vi "Pulse Generator 2.vi"() -> ()   [LabVIEW 2012]
uses:
  <vilib>/DAQmx/read.llb/DAQmx Read (Digital 1D Bool 1Chan 1Samp).vi
  <vilib>/DAQmx/create/channels.llb/DAQmx Create Channel (DI-Digital Input).vi
  <vilib>/DAQmx/miscellaneous.llb/DAQmx Fill In Error Info.vi
  <vilib>/Utility/file.llb/Write To Spreadsheet File (DBL).vi
panel:
  out "Track":bool=TRUE
  in  "ref?":bool=TRUE
  in  "load":bool
  in  "MW Delay":dbl=5e-08
  in  "Sig/Ref pause":dbl=7e-07
  in  "Tab Control":T1(tab)=enum."FLIM"
  in  "Rate (Hz)":dbl=1000.0
  in  "Pulse MW":bool=TRUE
  in  "Pulse Laser":bool
  in  "Delay Blocks":u16=4
  in  "Divide By":u16(ring) items=["1", "8", "16", "32"]
  in  "MW width Min":dbl=2e-08
  in  "MW width step size":dbl=5e-09
  in  "MW width Max":dbl=5e-07
  in  "Tau step size":dbl
  in  "Tau max":dbl
  in  "Tau min":dbl
  in  "Rabi Frequency":dbl
  in  "Pulse offset 2":dbl
  in  "Rabi Frequency":dbl
  in  "Tau max":dbl
  in  "Tau min":dbl
  in  "Tau step size":dbl
  in  "Equal Pulse length":bool
  in  "Pulse offset":dbl
  in  "Tau":dbl
  in  "Rabi Frequency  2":dbl
  in  "Tau' max 2":dbl
  in  "Tau' min 2":dbl
  in  "Tau' step size 2":dbl
  in  "Rabi Frequency":dbl
  in  "Tau min":dbl
  in  "Tau max":dbl
  in  "Tau step size":dbl
  in  "No. Pi Pulses":i32
  in  "Pulse offset":dbl
  in  "0->+?":bool
  in  "AOM Rest time":dbl=2e-06
  in  "Signal delay":dbl=1.1e-06
  in  "N Loop":i32=10000
  in  "APD signal width":dbl=5e-07
  out "Run":bool=TRUE
  out "Scan size":i32
  in  "file path (dialog if empty)":path=path "C:/Users/Ouyang Group/Documents/Data/12-5-13/current"
  in  "AOM Pulse length":dbl=2e-06
  in  "Path to spinapi.dll":path=path "C:/SpinCore/SpinAPI/dll/spinapi64.dll"
  in  "stop":bool
  in  "start/restart":bool
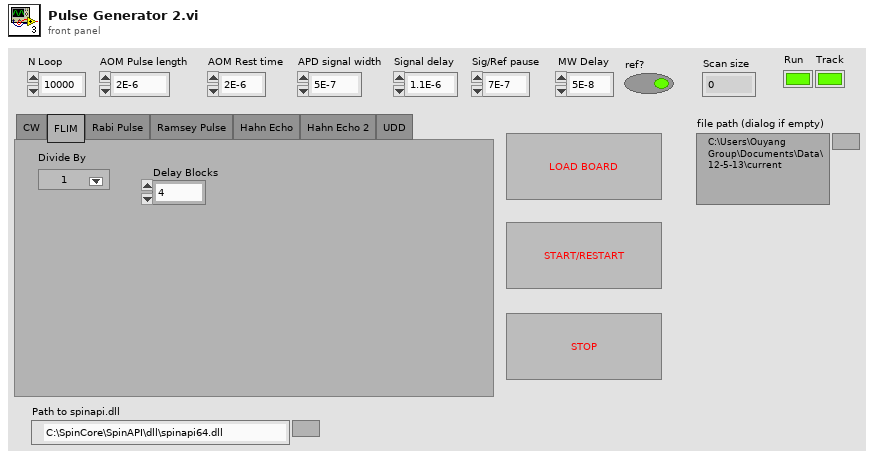
[diagram p1: front panel]
types:
  T1 = enum32{"CW", "FLIM", "Rabi Pulse", "Ramsey Pulse", "Hahn Echo", "Hahn Echo 2", "UDD"}
  T2 = enum16{"Pulse Program", "Frequency Registers", "TX Phase Registers", "RX Phase Registers"}
  T3 = cluster{"Instruct Data":i32, "Op Code":i32, "Flags":bool[], "Comments":string, "Time (s)":dbl}
  T4 = cluster{"Instruct Data":i32, "Op Code":i32, "Flags":bool[], "Comments":string, "Time (s)":dbl}[]
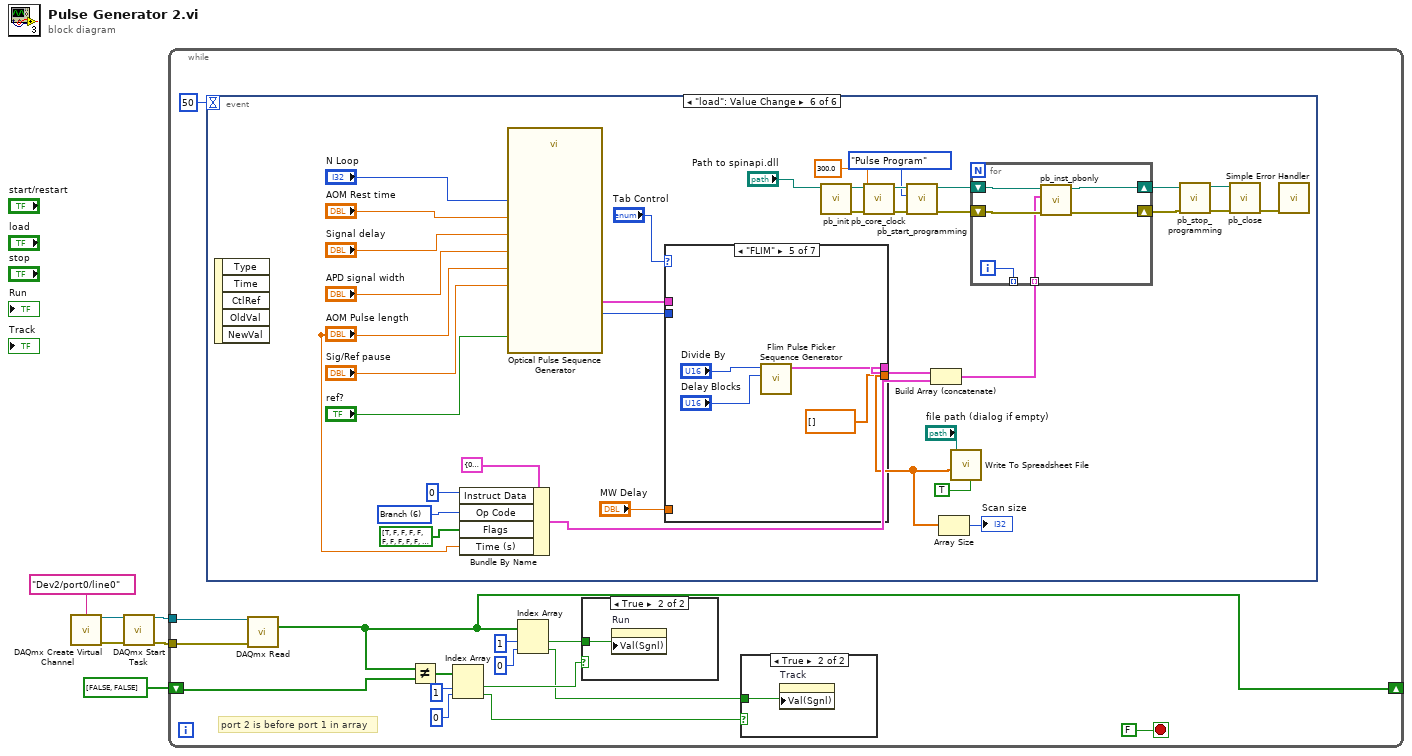
[diagram p0: block diagram]
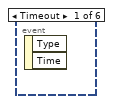
[diagram p3: hidden frame]
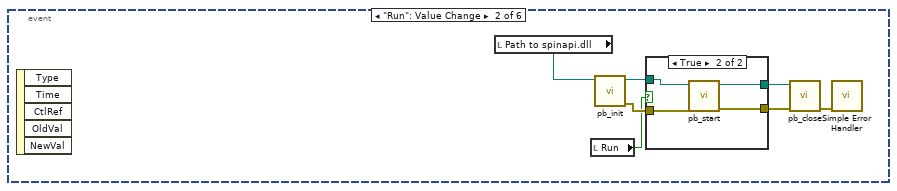
[diagram p4: hidden frame]
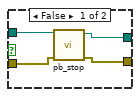
[diagram p5: hidden frame]
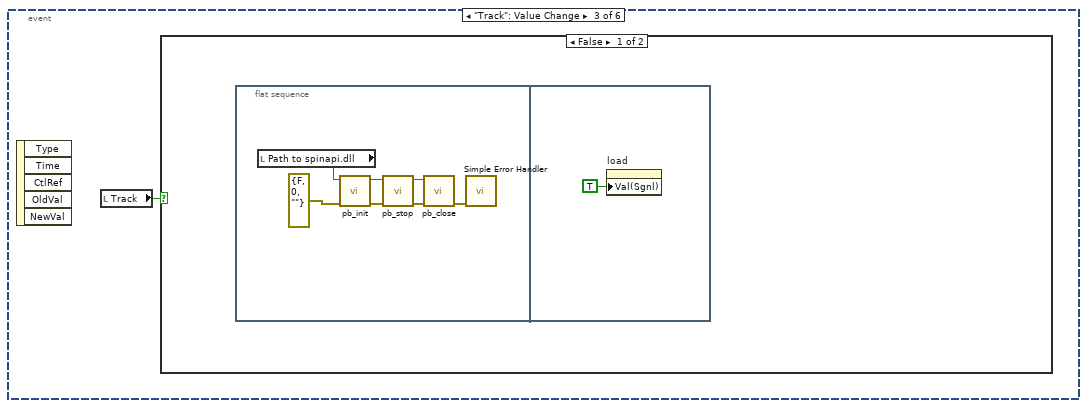
[diagram p6: hidden frame]
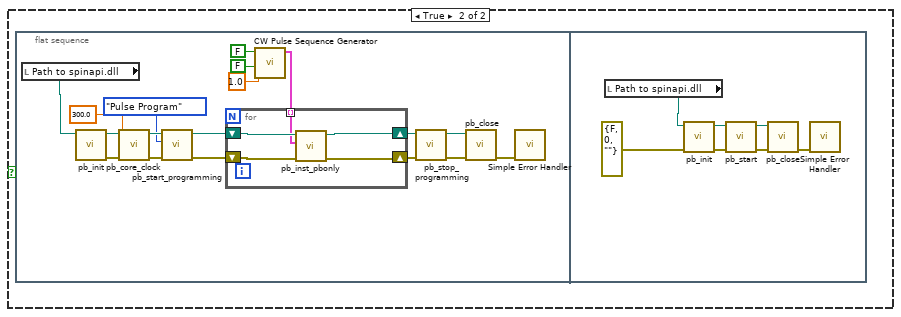
[diagram p7: hidden frame]
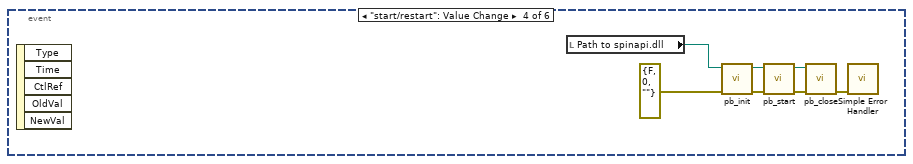
[diagram p8: hidden frame]
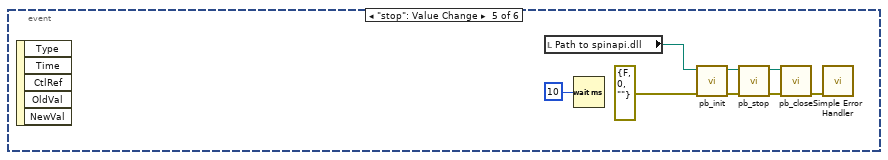
[diagram p9: hidden frame]
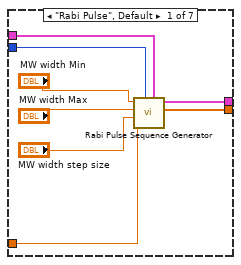
[diagram p10: hidden frame]
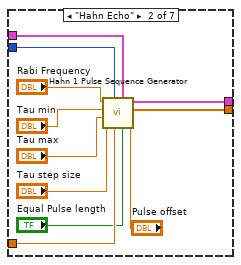
[diagram p11: hidden frame]
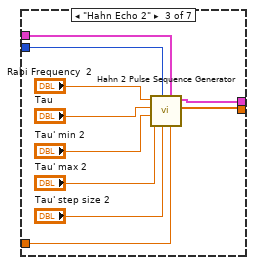
[diagram p12: hidden frame]
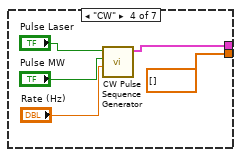
[diagram p13: hidden frame]
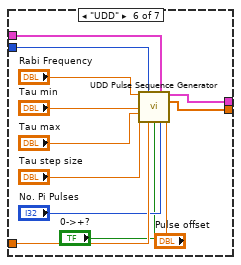
[diagram p14: hidden frame]
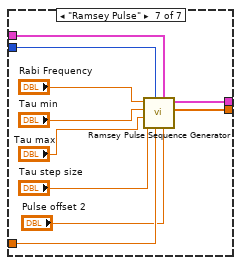
[diagram p15: hidden frame]
diagram:
  n1 = call-poly <vilib>:"DAQmx Create Virtual Channel.vi"("lines"=tag "Dev2/port0/line0") -> ("task out"=w3:refnum<k21>, "error out"=w2:errorcluster)  [unwired: 13 in]
  n2 = call <vilib>:"DAQmx Start Task.vi"("task/channels in"=w3, "error in"=w2) -> ("task out"=w4:refnum<k21>, "error out"=w5:errorcluster)  [unwired: 12 in]
  n3 = while {
    tunnel: w4 -> [w21]
    tunnel: w5 -> [w20]
    shift-right: [w9] -> _
    shift-left: bool[] [FALSE, FALSE] ("y") -> [w17]
    stop <- FALSE stop-if-true
    # "port 2 is before port 1 in array"
    n4 = event shown="[5] \"load\": Value Change" {
      selector: _ -> [_ _ _ _ _ _]
      dyn-events: _ -> [_ _ _ _ _ _]
      timeout: 50 -> [_ _ _ _ _ _]
      event Timeout {
        n5 = event-data() -> ()  [unwired: 1 in, 2 out]
      }
      event "Run": Value Change {
        n6 = event-data() -> ()  [unwired: 1 in, 5 out]
        n7 = local read "Path to spinapi.dll"() -> (w23:path)
        n8 = local read "Run"() -> (w27:bool)
        n9 = call "pb_init.vi"("path in"=w23) -> ("error out"=w28:errorcluster, "path out"=w29:path)  [unwired: 2 in, 7 out]
        n10 = case shown="True" w27 {
          tunnel: w29 -> [w33 w37]
          tunnel: w28 -> [w32 w36]
          tunnel: [w31 w35] -> w25
          tunnel: [w30 w34] -> w24
          frame False {
            n11 = call "pb_stop.vi"("error in (no error)"=w32, "path in"=w33) -> ("error out"=w30:errorcluster, "path out"=w31:path)  [unwired: 8 out]
          }
          frame True {
            n12 = call "pb_start.vi"("error in (no error)"=w36, "path in"=w37) -> ("error out"=w34:errorcluster, "path out"=w35:path)  [unwired: 1 in, 7 out]
          }
        }
        n13 = call "pb_close.vi"("error in (no error)"=w24, "path in"=w25) -> ("error out"=w26:errorcluster)  [unwired: 9 out]
        n14 = call <vilib>:"Simple Error Handler.vi"("error in (no error)"=w26) -> ()  [unwired: 1 in, 8 out]
      }
      event "Track": Value Change {
        n15 = event-data() -> ()  [unwired: 1 in, 5 out]
        n16 = local read "Track"() -> (w38:bool)
        n17 = case shown="False" w38 {
          frame False {
            n18 = flat-sequence {
              frame #0 {
                n19 = local read "Path to spinapi.dll"() -> (w39:path)
                n20 = call "pb_init.vi"("error in (no error)"=errorcluster {"status"=FALSE, "code"=0, "source"=""}, "path in"=w39) -> ("error out"=w41:errorcluster, "path out"=w43:path)  [unwired: 1 in, 7 out]
                n21 = call "pb_stop.vi"("error in (no error)"=w41, "path in"=w43) -> ("error out"=w40:errorcluster, "path out"=w42:path)  [unwired: 8 out]
                n22 = call "pb_close.vi"("error in (no error)"=w40, "path in"=w42) -> ("error out"=w45:errorcluster)  [unwired: 9 out]
                n23 = call <vilib>:"Simple Error Handler.vi"("error in (no error)"=w45) -> ()  [unwired: 1 in, 8 out]
              }
              frame #1 {
                n24 = property on="load" class="Bool (strict)"("Val(Sgnl)"=TRUE ("Value (Signaling)")) -> ()  [unwired: 2 in, 2 out]
              }
            }
          }
          frame True {
            n25 = flat-sequence {
              frame #0 {
                n26 = local read "Path to spinapi.dll"() -> (w47:path)
                n27 = call "pb_init.vi"("path in"=w47) -> ("error out"=w57:errorcluster, "path out"=w55:path)  [unwired: 3 in, 6 out]
                n28 = call "pb_core_clock.vi"("error in (no error)"=w57, "clock_freq (MHz)"=300.0, "path in"=w55) -> ("error out"=w58:errorcluster, "path out"=w56:path)  [unwired: 7 in]
                n29 = call "pb_start_programming.vi"("error in (no error)"=w58, "Device"=T2."Pulse Program", "path in"=w56) -> ("error out"=w61:errorcluster, "path out"=w60:path)  [unwired: 1 in, 6 out]
                n30 = call "CW Pulse Sequence Generator.vi"("Pulse Laser"=FALSE, "Pulse MW"=FALSE, "Rate (Hz)"=1.0) -> ("Pulse Sequence Out"=w51:T4)  [unwired: 7 in]
                n31 = for {
                  shift-right: [w67] -> w62
                  shift-left: w60 -> [w69]
                  shift-right: [w66] -> w63
                  shift-left: w61 -> [w68]
                  tunnel: w51 -> [w65] mode=indexing
                  n32 = call "pb_inst_pbonly.vi"("error in (no error)"=w68, "PB Instruction"=w65, "path in"=w69) -> ("error out"=w66:errorcluster, "path out"=w67:path)  [unwired: 2 in, 5 out]
                }
                n33 = call "pb_stop_programming.vi"("error in (no error)"=w63, "path in"=w62) -> ("error out"=w54:errorcluster, "path out"=w53:path)  [unwired: 1 in, 7 out]
                n34 = call "pb_close.vi"("error in (no error)"=w54, "path in"=w53) -> ("error out"=w64:errorcluster)  [unwired: 9 out]
                n35 = call <vilib>:"Simple Error Handler.vi"("error in (no error)"=w64) -> ()  [unwired: 1 in, 8 out]
              }
              frame #1 {
                n36 = local read "Path to spinapi.dll"() -> (w70:path)
                n37 = call "pb_init.vi"("error in (no error)"=errorcluster {"status"=FALSE, "code"=0, "source"=""}, "path in"=w70) -> ("error out"=w74:errorcluster, "path out"=w72:path)  [unwired: 1 in, 7 out]
                n38 = call "pb_start.vi"("error in (no error)"=w74, "path in"=w72) -> ("error out"=w75:errorcluster, "path out"=w71:path)  [unwired: 1 in, 7 out]
                n39 = call "pb_close.vi"("error in (no error)"=w75, "path in"=w71) -> ("error out"=w76:errorcluster)  [unwired: 9 out]
                n40 = call <vilib>:"Simple Error Handler.vi"("error in (no error)"=w76) -> ()  [unwired: 1 in, 8 out]
              }
            }
          }
        }
      }
      event "start/restart": Value Change {
        n41 = event-data() -> ()  [unwired: 1 in, 5 out]
        n42 = local read "Path to spinapi.dll"() -> (w83:path)
        n43 = call "pb_init.vi"("error in (no error)"=errorcluster {"status"=FALSE, "code"=0, "source"=""}, "path in"=w83) -> ("error out"=w80:errorcluster, "path out"=w78:path)  [unwired: 1 in, 7 out]
        n44 = call "pb_start.vi"("error in (no error)"=w80, "path in"=w78) -> ("error out"=w81:errorcluster, "path out"=w77:path)  [unwired: 1 in, 7 out]
        n45 = call "pb_close.vi"("error in (no error)"=w81, "path in"=w77) -> ("error out"=w82:errorcluster)  [unwired: 9 out]
        n46 = call <vilib>:"Simple Error Handler.vi"("error in (no error)"=w82) -> ()  [unwired: 1 in, 8 out]
      }
      event "stop": Value Change {
        n47 = event-data() -> ()  [unwired: 1 in, 5 out]
        n48 = local read "Path to spinapi.dll"() -> (w90:path)
        n49 = Wait (ms)(milliseconds to wait=u32 10) -> ()  [unwired: 1 out]
        n50 = call "pb_init.vi"("error in (no error)"=errorcluster {"status"=FALSE, "code"=0, "source"=""}, "path in"=w90) -> ("error out"=w87:errorcluster, "path out"=w85:path)  [unwired: 1 in, 7 out]
        n51 = call "pb_stop.vi"("error in (no error)"=w87, "path in"=w85) -> ("error out"=w88:errorcluster, "path out"=w84:path)  [unwired: 8 out]
        n52 = call "pb_close.vi"("error in (no error)"=w88, "path in"=w84) -> ("error out"=w89:errorcluster)  [unwired: 9 out]
        n53 = call <vilib>:"Simple Error Handler.vi"("error in (no error)"=w89) -> ()  [unwired: 1 in, 8 out]
      }
      event "load": Value Change {
        w115 = 6 items=["Continue", "Stop", "Loop", "End Loop", "JSR", "RTS", "Branch", "Long Delay", "Wait"] ("Op Code")
        n54 = event-data() -> ()  [unwired: 1 in, 5 out]
        n55 = Bundle By Name(cluster=T3 {"Instruct Data"=0, "Op Code"=0, "Flags"=[FALSE, FALSE, FALSE, FALSE, FALSE, FALSE, FALSE, FALSE, FALSE, FALSE, FALSE, FALSE, FALSE, FALSE, FALSE, FALSE, FALSE, FALSE, FALSE, FALSE, FALSE, TRUE, TRUE, TRUE], "Comments"="", "Time (s)"=0.01} ("PB Inst 2"), "Instruct Data"=0, "Op Code"=w115, "Flags"=bool[] [TRUE, FALSE, FALSE, FALSE, FALSE, FALSE, FALSE, FALSE, FALSE, FALSE, FALSE, FALSE, FALSE, FALSE, FALSE, FALSE, FALSE, FALSE, FALSE, FALSE, FALSE, TRUE, TRUE, TRUE], "Time (s)"="AOM Pulse length") -> (w127:T3)
        n56 = call "Optical Pulse Sequence Generator.vi"("ref?"="ref?", "N Loop"="N Loop", "Sig/Ref pause"="Sig/Ref pause", "AOM Rest time"="AOM Rest time", "Signal delay"="Signal delay", "APD signal width"="APD signal width", "AOM Pulse length"="AOM Pulse length") -> ("Array"=w122:T4, "No. Instructions"=w123:i32)  [unwired: 3 in]
        n57 = case shown="\"FLIM\"" "Tab Control" {
          tunnel: w122 -> [w130 w140 w149 _ _ w176 w185]
          tunnel: w123 -> [w131 w141 w150 _ _ w177 w184]
          tunnel: "MW Delay" -> [w132 w142 w151 _ _ w169 w179]
          tunnel: [w129 w139 w148 w158 w165 w175 w186] -> w126
          tunnel: [w128 w138 w147 dbl[] [] ("Tau") dbl[] [] ("Tau") w174 w187] -> w113
          frame "Rabi Pulse", Default {
            n58 = call "Rabi Pulse Sequence Generator.vi"("Optical Pulse"=w130, "No. Instructions"=w131, "MW Delay"=w132, "MW width step size"="MW width step size", "MW width Max"="MW width Max", "MW width Min"="MW width Min") -> ("Pulse Width"=w128:dbl[], "Pulse Sequence Out"=w129:T4)  [unwired: 4 in]
          }
          frame "Hahn Echo" {
            n59 = call "Hahn 1 Pulse Sequence Generator.vi"("Pulse offset"="Pulse offset", "Equal Pulse length"="Equal Pulse length", "Array"=w140, "MW Delay"=w142, "No. Instructions"=w141, "Tau step size"="Tau step size", "Tau max"="Tau max", "Tau min"="Tau min", "Rabi Frequency"="Rabi Frequency") -> ("Tau"=w138:dbl[], "Pulse Sequence"=w139:T4)  [unwired: 1 in]
          }
          frame "Hahn Echo 2" {
            n60 = call "Hahn 2 Pulse Sequence Generator.vi"("MW Delay"=w151, "Optical Pulse Sequence"=w149, "Tau' step size 2"="Tau' step size 2", "No. Instructions"=w150, "Tau' max 2"="Tau' max 2", "Tau' min 2"="Tau' min 2", "Tau"="Tau", "Rabi Frequency  2"="Rabi Frequency  2") -> ("Tau'"=w147:dbl[], "Pulse Sequence"=w148:T4)  [unwired: 2 in]
          }
          frame "CW" {
            n61 = call "CW Pulse Sequence Generator.vi"("Pulse Laser"="Pulse Laser", "Pulse MW"="Pulse MW", "Rate (Hz)"="Rate (Hz)") -> ("Pulse Sequence Out"=w158:T4)  [unwired: 7 in]
          }
          frame "FLIM" {
            n62 = call "Flim Pulse Picker Sequence Generator.vi"("Delay Blocks"="Delay Blocks", "Divide By"="Divide By") -> ("Pulse Sequence Out"=w165:T4)  [unwired: 9 in]
          }
          frame "UDD" {
            n63 = call "UDD Pulse Sequence Generator.vi"("Rabi Frequency"="Rabi Frequency", "No. Instructions"=w177, "Array"=w176, "Tau min"="Tau min", "Tau max"="Tau max", "Tau step size"="Tau step size", "MW Delay"=w169, "0->+?"="0->+?", "No. Pi Pulses"="No. Pi Pulses", "Pulse offset"="Pulse offset") -> ("Pulse Sequence"=w175:T4, "Tau"=w174:dbl[])  [unwired: 4 in]
          }
          frame "Ramsey Pulse" {
            n64 = call "Ramsey Pulse Sequence Generator.vi"("Pulse offset"="Pulse offset 2", "Array"=w185, "MW Delay"=w179, "No. Instructions"=w184, "Tau step size"="Tau step size", "Tau max"="Tau max", "Tau min"="Tau min", "Rabi Frequency"="Rabi Frequency") -> ("Tau"=w187:dbl[], "Pulse Sequence"=w186:T4)  [unwired: 2 in]
          }
        }
        n65 = call "pb_init.vi"("path in"="Path to spinapi.dll") -> ("error out"=w100:errorcluster, "path out"=w98:path)  [unwired: 3 in, 6 out]
        n66 = call "pb_core_clock.vi"("error in (no error)"=w100, "clock_freq (MHz)"=300.0, "path in"=w98) -> ("error out"=w101:errorcluster, "path out"=w99:path)  [unwired: 7 in]
        n67 = call "pb_start_programming.vi"("error in (no error)"=w101, "Device"=T2."Pulse Program", "path in"=w99) -> ("error out"=w104:errorcluster, "path out"=w103:path)  [unwired: 1 in, 6 out]
        n68 = Build Array (concatenate)(w126, w127) -> (w112:T4)
        n69 = Array Size(array=w113) -> (size(s)=→"Scan size":i32)
        n70 = call-poly <vilib>:"Write To Spreadsheet File.vi"("transpose? (no:F)"=TRUE, "1D data"=w113, "file path (dialog if empty)"="file path (dialog if empty)") -> ()  [unwired: 5 in, 1 out]
        n71 = for {
          shift-right: [w191] -> w105
          shift-left: w103 -> [w193]
          shift-right: [w190] -> w106
          shift-left: w104 -> [w192]
          tunnel: [w189] -> _ mode=indexing
          tunnel: w112 -> [w188] mode=indexing
          i -> [w189]
          n72 = call "pb_inst_pbonly.vi"("error in (no error)"=w192, "PB Instruction"=w188, "path in"=w193) -> ("error out"=w190:errorcluster, "path out"=w191:path)  [unwired: 2 in, 5 out]
        }
        n73 = call "pb_stop_programming.vi"("error in (no error)"=w106, "path in"=w105) -> ("error out"=w97:errorcluster, "path out"=w96:path)  [unwired: 1 in, 7 out]
        n74 = call "pb_close.vi"("error in (no error)"=w97, "path in"=w96) -> ("error out"=w108:errorcluster)  [unwired: 9 out]
        n75 = call <vilib>:"Simple Error Handler.vi"("error in (no error)"=w108) -> ()  [unwired: 1 in, 8 out]
      }
    }
    n76 = call-poly <vilib>:"DAQmx Read.vi"("task/channels in"=w21, "error in"=w20) -> ("data"=w9:bool[])  [unwired: 11 in, 2 out]
    n77 = Not Equal?(x=w9, y=w17) -> (x != y?=w16:bool[])
    n78 = Index Array(array=w16, index #1=1 ("index"), index #2=0 ("index")) -> (element #1=w14:bool, element #2=w11:bool)
    n79 = Index Array(array=w9, index #1=1 ("index"), index #2=0 ("index")) -> (element #1=w12:bool, element #2=w10:bool)
    n80 = case shown="True" w14 {
      tunnel: w12 -> [_ w194]
      frame False {
      }
      frame True {
        n81 = property on="Run" class="Bool (strict)"("Val(Sgnl)"=w194) -> ()  [unwired: 2 in, 2 out]
      }
    }
    n82 = case shown="True" w11 {
      tunnel: w10 -> [_ w22]
      frame False {
      }
      frame True {
        n83 = property on="Track" class="Bool (strict)"("Val(Sgnl)"=w22) -> ()  [unwired: 2 in, 2 out]
      }
    }
  }
